vi "Read Original Settings File.vi"(8 "Error In":errorcluster, 11 "Original Settings Filepath":path) -> (0 "Error Out":errorcluster, 3 "Settings File Contents":string)   [LabVIEW 2023, in "Error Manager.lvlib" / "Settings.lvclass"]
doc: "This VI reads the contents of the settings file.\n\nIn this VI, the settings file is referred to as the \"Original Settings File\", to distinguish it from the \"Temporary Settings File\", which is a temporary file.\n\nThe settings file is accessed using read-only access, ensuring that the original settings file is not modified."
uses:
  Settings.lvclass
  Settings.lvclass/Settings.ctl
panel:
  # "Development\nControls or indicators that are useful for development or testing, but which are not outputs of the VI."
  # "Input\nInputs to the VI"
  # "Output\nOutputs of the VI"
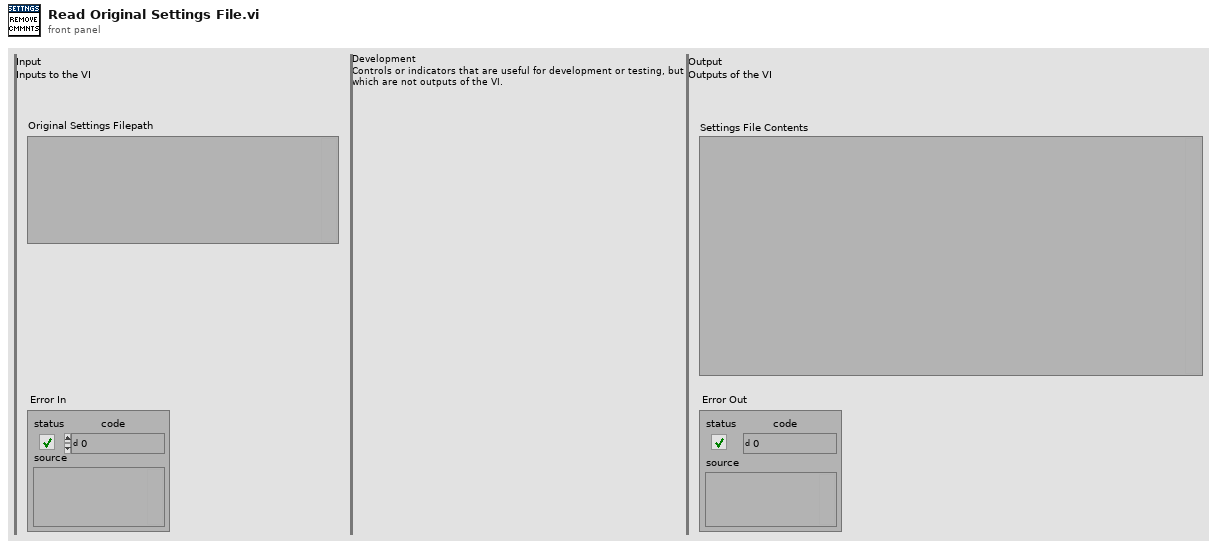
[diagram p1: front panel]
types:
  T1 = enum16{"open", "replace", "create", "open or create", "replace or create", "replace or create with confirmation"}
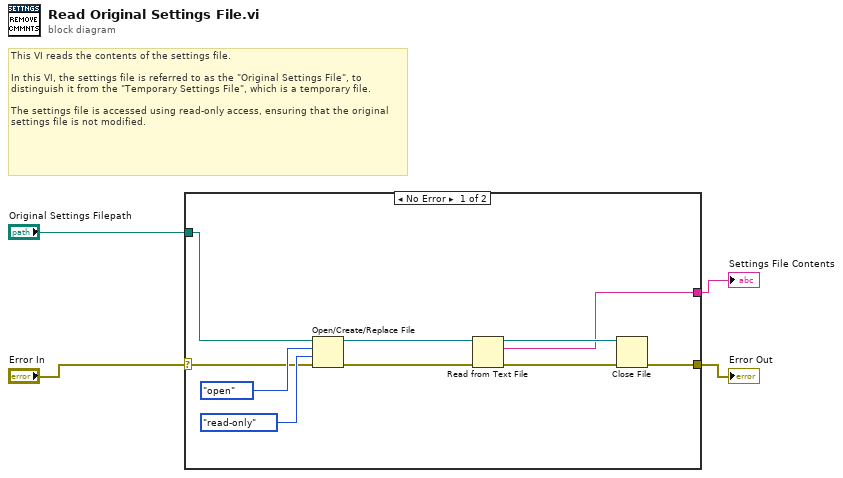
[diagram p0: block diagram]
diagram:
  # "This VI reads the contents of the settings file.\n\nIn this VI, the settings file is referred to as the \"Original Settings File\", to distinguish it from the \"Temporary Settings File\", which is a temporary file.\n\nThe settings file is accessed using read-only access, ensuring that the original settings file is not modified."
  n1 = case shown="No Error" "Error In" {
    selector: "Error In" -> [w10 w15]
    tunnel: [w6 w15] -> w3
    tunnel: "Original Settings Filepath" -> [w9 _]
    tunnel: [w5 _] -> w1
    frame No Error {
      n2 = Open/Create/Replace File(file path (use dialog)=w9, error in=w10, operation (0:open)=T1."open", access (0:read/write)=enum16{"read/write", "read-only", "write-only"}."read-only") -> (refnum out=w11:refnum<file>, error out=w12:errorcluster)  [unwired: 2 in, 1 out]
      n3 = Read from Text File(file (use dialog)=w11, error in=w12) -> (refnum out=w7:refnum<file>, text=w5:string, error out=w8:errorcluster)  [unwired: 2 in, 1 out]
      n4 = Close File(refnum=w7, error in=w8) -> (error out=w6:errorcluster)  [unwired: 1 out]
    }
    frame Error {
    }
  }
  "Error Out" <- w3
  "Settings File Contents" <- w1
